vi "Insert Subroutine.vi"(0 "Test Executive Ref":refnum<data-value>, 1 "Parent ID":string, 5 "Name":string, 9 "Subroutine Path":string, 11 "error in (no error)":errorcluster, 12 "Insertion Index":i32=-1, 13 "Path Builder":refnum<class "IPath Builder.lvclass">, 14 "Persistence":refnum<class "IPersist.lvclass">) -> (3 "Unique ID out":string, 4 "Test Executive Ref out":refnum<data-value>, 8 "Replaced?":bool, 15 "error out":errorcluster)   [LabVIEW 2019, in "Test Executive.lvlib" / "TestExecutive Ref.lvclass"]
uses:
  <vilib>/gpm_packages/@cs/test-executive/Source/Test Executive/TestExecutive Ref/TestExecutive Ref.lvclass
  <vilib>/gpm_packages/@cs/test-executive/Source/Test Executive/ITestExecutive/ITest Executive.lvclass
  <vilib>/gpm_packages/@cs/persistence/source/IPersist/IPersist.lvclass
  <vilib>/gpm_packages/@cs/test-executive/Source/Path Builder/IPath Builder/IPath Builder.lvclass
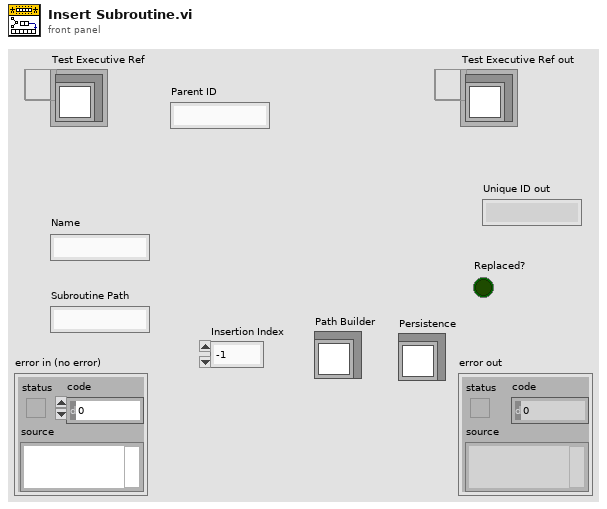
[diagram p1: front panel]
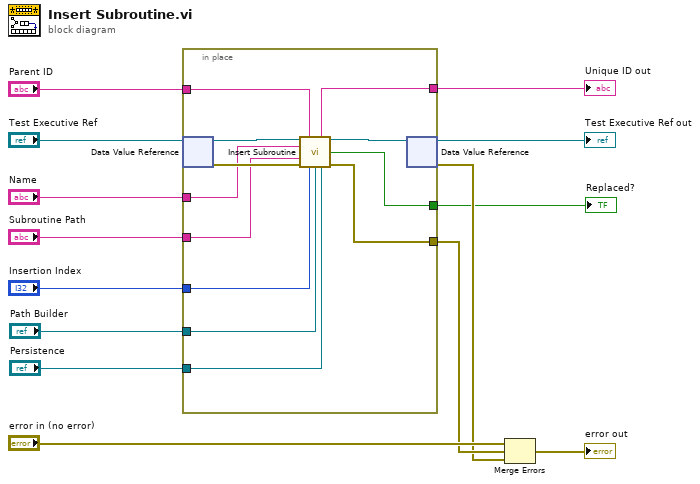
[diagram p0: block diagram]
diagram:
  n1 = in-place {
    in-place-border: "Parent ID" -> [w22]
    in-place-border: "Name" -> [w20]
    in-place-border: "Subroutine Path" -> [w19]
    in-place-border: "Insertion Index" -> [w21]
    in-place-border: [w18] -> w8
    in-place-border: [w23] -> w6
    in-place-border: "Persistence" -> [w17]
    in-place-border: "Path Builder" -> [w16]
    in-place-border: [w15] -> w1
    n2 = in-place-dvr #1("Test Executive Ref") -> (w26:refnum<class "ITest Executive.lvclass">, w25:errorcluster)
    n3 = call-dynamic "Insert Subroutine.vi"("ITest Executive in"=w26, "Parent ID"=w22, "Name"=w20, "File Path"=w19, "error in (no error)"=w25, "Insertion Index"=w21, "Path Builder"=w16, "Persistence"=w17) -> ("Unique ID out"=w18:string, "ITest Executive out"=w24:refnum<class "ITest Executive.lvclass">, "Replaced?"=w15:bool, "error out"=w23:errorcluster)  [unwired: 4 in]
    n4 = in-place-dvr #1(w24) -> (→"Test Executive Ref out":refnum<data-value>, w5:errorcluster)
  }
  "Unique ID out" <- w8
  "Replaced?" <- w1
  n5 = Merge Errors("error in (no error)", w6, w5) -> (→"error out":errorcluster)
